vi "FDR Def_Start_Results.vi"(0 "System no.":i32=1 min=1 step=1, 1 "Board":i32=1 min=1 max=5 step=1, 2 "Routinename":string, 3 "Scan axis settings":T7={"Scan axis"="", "Range scan axis"=0.1, "Set Mid. pos?"=FALSE, "Mid. pos. scan axis"=0.1} {"Mid. pos. scan axis" format="%.4f"; "Range scan axis" format="%.4f"}, 4 "Step axis settings":T6={"Step axis"="", "Range step axis"=0.1, "Set Mid. pos?"=FALSE, "Mid. pos. step axis"=0.1} {"Mid. pos. step axis" format="%.4f"; "Range step axis" format="%.4f"}, 5 "error in":errorcluster, 6 "Treshold level":dbl=1.0 format="%.3f", 7 "Frequency settings":cluster{"Set frequency?":bool, "Frequency":dbl}={"Set frequency?"=FALSE, "Frequency"=10.0} {"Frequency" format="%.3f"}, 8 "Velocity settings":cluster{"Set velocity?":bool, "Velocity":dbl}={"Set velocity?"=FALSE, "Velocity"=0.1} {"Velocity" format="%.4f"}, 9 "Stop position option settings":T5, 12 "Stop refnum":refnum<vi>, 13 "Polling time in ms":u32=1) -> (14 "Scan successful?":bool, 15 "Level at max. pos.":dbl=1.0 format="%.4f", 16 "Pos. at max. information":string, 19 "error out":errorcluster)   [LabVIEW 2026]
doc: "Defines a fast alignment area scan routine, starts scan, waits until scan has finished and queries results. If Stop refnum or Local stop is TRUE, VI sends #24 and stops."
panel:
  in  "Max. relative input level (MAIL) settings":T1={"Set max. input level?"=FALSE, "MAIL"=80.0}
  in  "Min. relative input level (MIIL) settings":T2={"Set min. input level?"=FALSE, "MIIL"=10.0}
  in  "Centroid method settings":T3
  in  "Target type settings":T4
  in  "Local stop":bool
  # "Defines fast raster scan, starts scan, waits until scan has finished and queries results.  If Stop refnum or\nLocal stop is TRUE, VI sends #24 and stops."
  # "If Yes:"
  # "If Yes:"
  # "If Yes:"
  # "If Yes:"
  # "If Yes:"
  # "If Yes:"
  # "If Yes:"
  # "If Yes:"
  # "If Yes:"
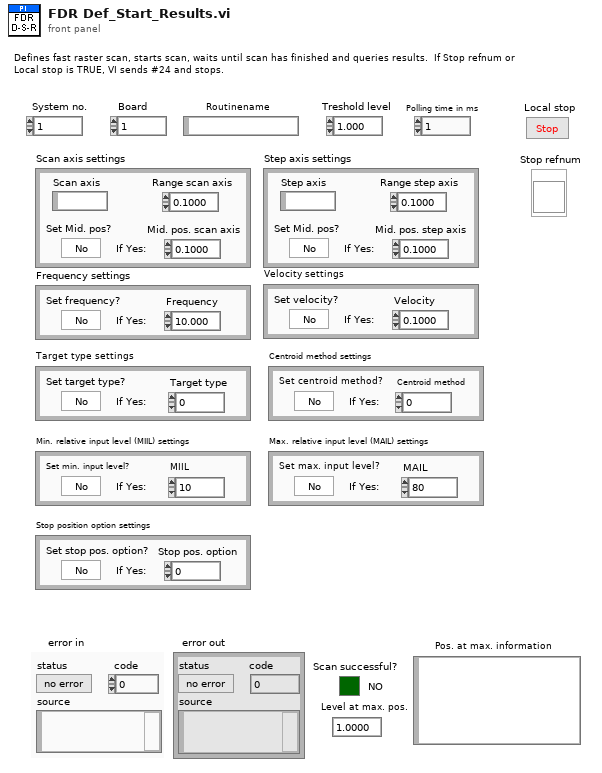
[diagram p1: front panel]
types:
  T1 = cluster{"Set max. input level?":bool, "MAIL":dbl}
  T2 = cluster{"Set min. input level?":bool, "MIIL":dbl}
  T3 = cluster{"Set centroid method?":bool, "Centroid method":i32}
  T4 = cluster{"Set target type?":bool, "Target type":i32}
  T5 = cluster{"Set stop pos. option?":bool, "Stop pos. option":i32}
  T6 = cluster{"Step axis":string, "Range step axis":dbl, "Set Mid. pos?":bool, "Mid. pos. step axis":dbl}
  T7 = cluster{"Scan axis":string, "Range scan axis":dbl, "Set Mid. pos?":bool, "Mid. pos. scan axis":dbl}
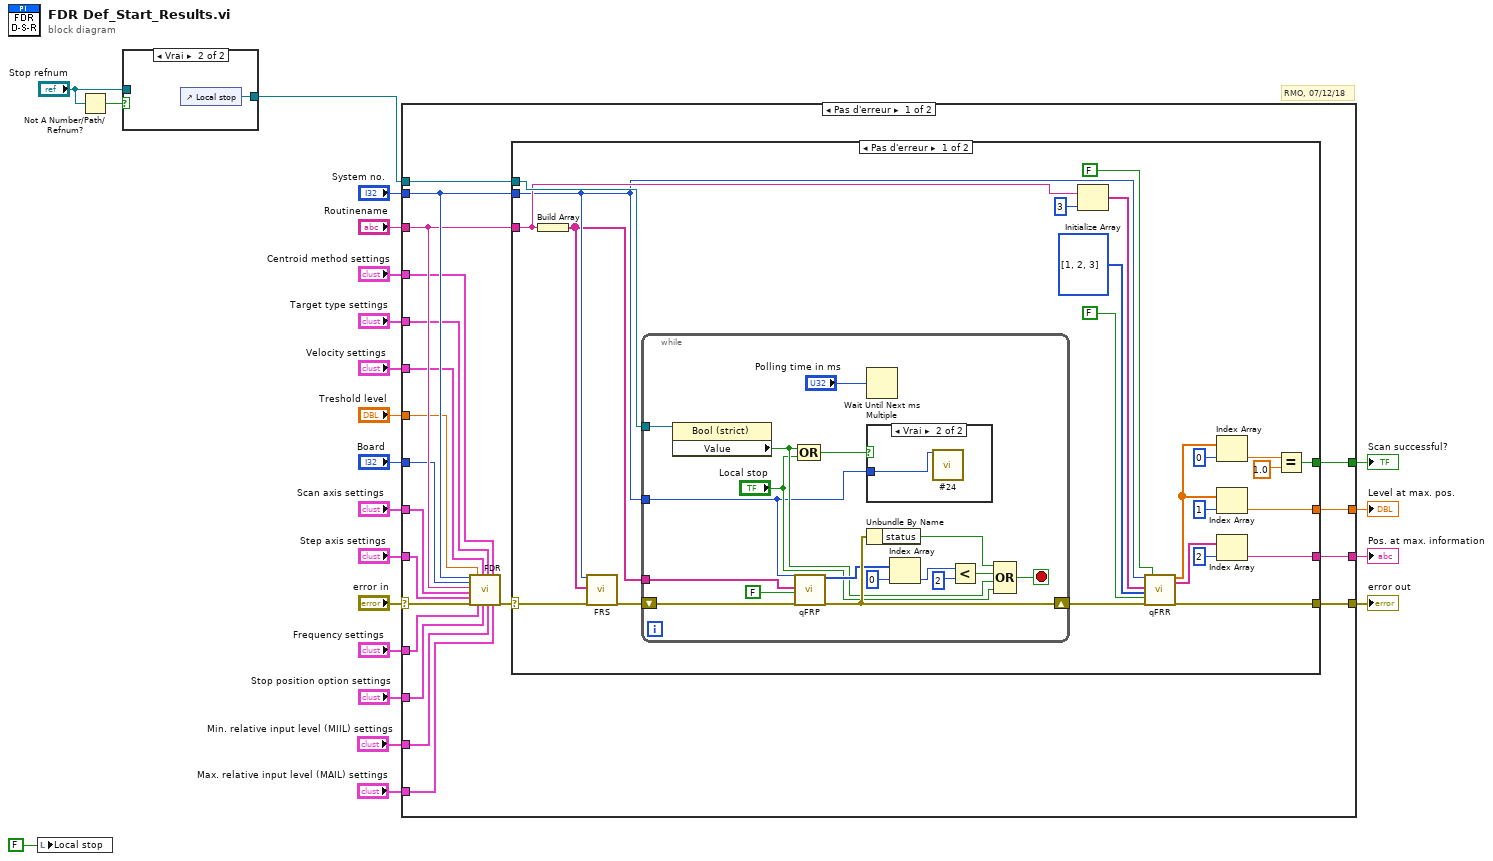
[diagram p0: block diagram]
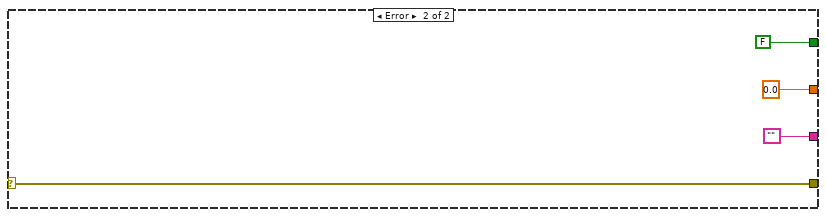
[diagram p4: hidden frame]
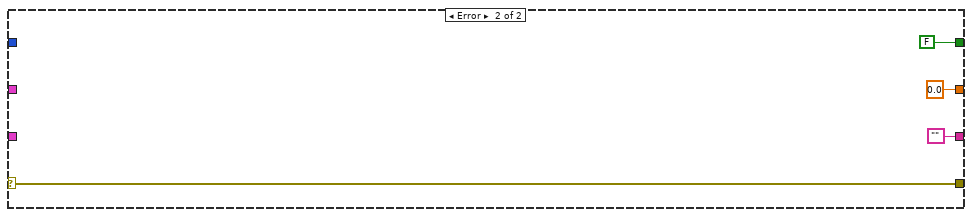
[diagram p5: hidden frame]
diagram:
  # "RMO, 07/12/18"
  n1 = local write "Local stop"(FALSE ("Local stop")) -> ()
  n2 = Not A Number/Path/Refnum?(number/path/refnum="Stop refnum") -> (NaN/Path/Refnum?=w18:bool)
  n3 = case shown="Vrai" w18 {
    tunnel: [w23 w24] -> w17
    tunnel: "Stop refnum" -> [w23 _]
    frame False {
    }
    frame True {
      n4 = control-ref of="Local stop"() -> (w24:refnum<vi>)
    }
  }
  n5 = case shown="Pas d'erreur" "error in" {
    selector: "error in" -> [w25 w90]
    tunnel: [w37 w90] -> w22
    tunnel: [w40 FALSE] -> w21
    tunnel: w17 -> [w43 _]
    tunnel: "System no." -> [w42 _]
    tunnel: "Routinename" -> [w41 _]
    tunnel: [w39 0.0 ("Numeric")] -> w14
    tunnel: [w38 "" ("String")] -> w13
    tunnel: "Board" -> [w36 _]
    tunnel: "Scan axis settings" -> [w35 _]
    tunnel: "Step axis settings" -> [w34 _]
    tunnel: "Frequency settings" -> [w33 _]
    tunnel: "Stop position option settings" -> [w32 _]
    tunnel: "Treshold level" -> [w31 _]
    tunnel: "Velocity settings" -> [w30 _]
    tunnel: "Target type settings" -> [w29 _]
    tunnel: "Centroid method settings" -> [w28 _]
    tunnel: "Min. relative input level (MIIL) settings" -> [w27 _]
    tunnel: "Max. relative input level (MAIL) settings" -> [w26 _]
    frame No Error {
      n6 = call "FDR.vi"("System no."=w42, "Board"=w36, "Routinename"=w41, "Scan axis settings"=w35, "Step axis settings"=w34, "error in"=w25, "Threshold level"=w31, "Frequency settings"=w33, "Velocity settings"=w30, "Stop position option settings"=w32, "Target type settings"=w29, "Min. relative input level (MIIL) settings"=w27, "Centroid method settings"=w28, "Max. relative input level (MAIL) settings"=w26) -> ("error out"=w44:errorcluster)  [unwired: 5 out]
      n7 = case shown="Pas d'erreur" w44 {
        selector: w44 -> [w48 w86]
        tunnel: w43 -> [w67 _]
        tunnel: w42 -> [w46 _]
        tunnel: w41 -> [w63 _]
        tunnel: [w56 FALSE] -> w40
        tunnel: [w54 0.0 ("Numeric")] -> w39
        tunnel: [w50 "" ("String")] -> w38
        tunnel: [w49 w86] -> w37
        frame No Error {
          n8 = Build Array(w63) -> (w45:string[])
          n9 = call "FRS.vi"("System no."=w46, "Routines to start"=w45, "error in"=w48) -> ("error out"=w47:errorcluster)  [unwired: 16 out]
          n10 = while {
            tunnel: w67 -> [w83]
            shift-right: [w80] -> w66
            shift-left: w47 -> [w82]
            tunnel: w46 -> [w69]
            tunnel: w45 -> [w73]
            stop <- w84 stop-if-true
            n11 = property class="Bool (strict)"(reference=w83) -> ("Value"=w72:bool)  [unwired: 1 in, 2 out]
            n12 = call "qFRP.vi"("System no."=w69, "Routines to query"=w73, "All routines?"=FALSE, "error in"=w82) -> ("Status"=w78:i32[], "error out"=w80:errorcluster)  [unwired: 14 out]
            n13 = Compound Arithmetic op=OR(w72, "Local stop") -> (w70:bool)
            n14 = Wait Until Next ms Multiple(millisecond multiple="Polling time in ms") -> ()  [unwired: 1 out]
            n15 = case shown="Vrai" w70 {
              tunnel: w69 -> [_ w85]
              frame False {
              }
              frame True {
                n16 = call "#24.vi"("System no."=w85) -> ()  [unwired: 1 in, 18 out]
              }
            }
            n17 = Unbundle By Name(w80) -> ("status"=w81:bool)
            n18 = Index Array(array=w78, index=0) -> (element=w76:i32)
            n19 = Less?(x=w76, y=2) -> (x < y?=w74:bool)
            n20 = Compound Arithmetic op=OR(w81, w74, w72, "Local stop") -> (w84:bool)
          }
          n21 = Initialize Array(w63, 3 ("dimension size")) -> (w61:string[])
          n22 = call "qFRR.vi"("System no."=w46, "Routinename"=w61, "ResultID"=i32[] [1, 2, 3], "Query all?"=FALSE, "error in"=w66, "Use FRH?"=FALSE) -> ("Value (num.)"=w55:dbl[], "Value (string)"=w51:string[], "error out"=w49:errorcluster)  [unwired: 11 out]
          n23 = Index Array(array=w55, index=0) -> (element=w58:dbl)
          n24 = Index Array(array=w55, index=1) -> (element=w54:dbl)
          n25 = Index Array(array=w51, index=2) -> (element=w50:string)
          n26 = Equal?(x=w58, y=1.0) -> (x = y?=w56:bool)
        }
        frame Error {
        }
      }
    }
    frame Error {
    }
  }
  "error out" <- w22
  "Scan successful?" <- w21
  "Level at max. pos." <- w14
  "Pos. at max. information" <- w13
